vi "Find and Replace.vi"(9 "Replacement":string, 10 "Find":string, 11 "Search String":string) -> (3 "Returned String":string)   [LabVIEW 2021]
doc: "Find all strings within and string and replace it with a given string. Returns the altered string."
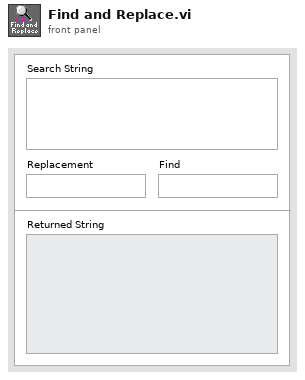
[diagram p1: front panel]
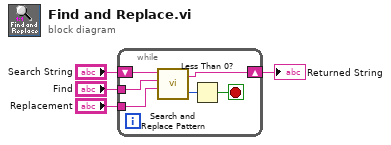
[diagram p0: block diagram]
diagram:
  n1 = while {
    shift-right: [w5] -> w1
    shift-left: "Search String" -> [w10]
    tunnel: "Find" -> [w9]
    tunnel: "Replacement" -> [w8]
    stop <- w6 stop-if-true
    n2 = call <vilib>:"Search and Replace Pattern.vi"("string"=w10, "regular expression (\"\")"=w9, "replace string (\"\")"=w8) -> ("result string"=w5:string, "offset past match"=w7:i32)  [unwired: 2 in]
    n3 = Less Than 0?(x=w7) -> (x < 0?=w6:bool)
  }
  "Returned String" <- w1
